vi "Subscribe to Roles.vi"(8 "error in (no error)":errorcluster, 11 "Module in":refnum<class "Module.lvclass">) -> (0 "error out":errorcluster, 3 "Module out":refnum<class "Module.lvclass">)   [LabVIEW 2020, in "Volatus.lvlib" / "Module.lvclass"]
uses:
  Module.lvclass
  Module.lvclass/Module.ctl
  VolatusAPI/VolatusAPI.lvclass
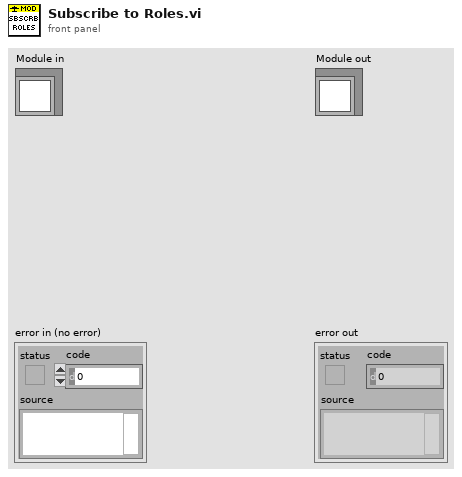
[diagram p1: front panel]
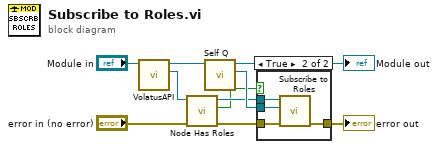
[diagram p0: block diagram]
diagram:
  n1 = call "VolatusAPI.vi"("Module in"="Module in") -> ("VolatusAPI"=w2:refnum<class "VolatusAPI.lvclass">, "Module out"=w6:refnum<class "Module.lvclass">)  [unwired: 9 in]
  n2 = call "Node Has Roles.vi"("error in (no error)"="error in (no error)", "VolatusAPI in"=w2) -> ("error out"=w4:errorcluster, "Node Has Roles"=w1:bool, "VolatusAPI out"=w3:refnum<class "VolatusAPI.lvclass">)  [unwired: 7 in]
  n3 = call "Self Q.vi"("Module in"=w6) -> ("Self Q"=w8:refnum<class "MessageQ.lvclass">, "Module out"=→"Module out":refnum<class "Module.lvclass">)  [unwired: 9 in]
  n4 = case shown="True" w1 {
    tunnel: w8 -> [_ w15]
    tunnel: [w11 w14] -> w7
    tunnel: w4 -> [w11 w13]
    tunnel: w3 -> [_ w12]
    frame False {
    }
    frame True {
      n5 = call "Subscribe to Roles.vi"("error in (no error)"=w13, "SelfQ"=w15, "VolatusAPI in"=w12) -> ("error out"=w14:errorcluster)  [unwired: 7 in, 1 out]
    }
  }
  "error out" <- w7
